vi "Main.vi"() -> ()   [LabVIEW 2017]
uses:
  Controles/Objetos.ctl
  <vilib>/addons/database/Connection.llb/Conn ObjectReference.ctl
  <vilib>/NI/AMC/Update Message Routing Info.vi
  <vilib>/NI/AMC/Create Multiple Messages.vi
  <vilib>/NI/AMC/Read Termination Message.vi
  <vilib>/NI/AMC/Create Single Message.vi
  <vilib>/NI/AMC/Send Message.vi
  <vilib>/NI/AMC/Globals.vi
  <vilib>/Utility/file.llb/Read Delimited Spreadsheet (string).vi
  Globals/Global.vi
  <vilib>/addons/database/Connection.llb/DB Tools Open Connec (Path).vi
  <vilib>/addons/database/_DB Variant To Data/Database Variant To Data.xnode
  <vilib>/addons/database/NI_Database_API.lvlib
  <vilib>/NI/AMC/AMC.lvlib
panel:
  out "BBDD":bool
  in  "Consulta":bool
  in  "Registrado":string
  in  "Cambiar de usuario":bool
  in  "Jiffy csv":path
  in  "Registrar":bool
  out "error out":errorcluster
  in  "Objetos":T1
  out "DataBase":bool
  # "Contabilizador"
  # "powered by"
  # "Contabilizador v01"
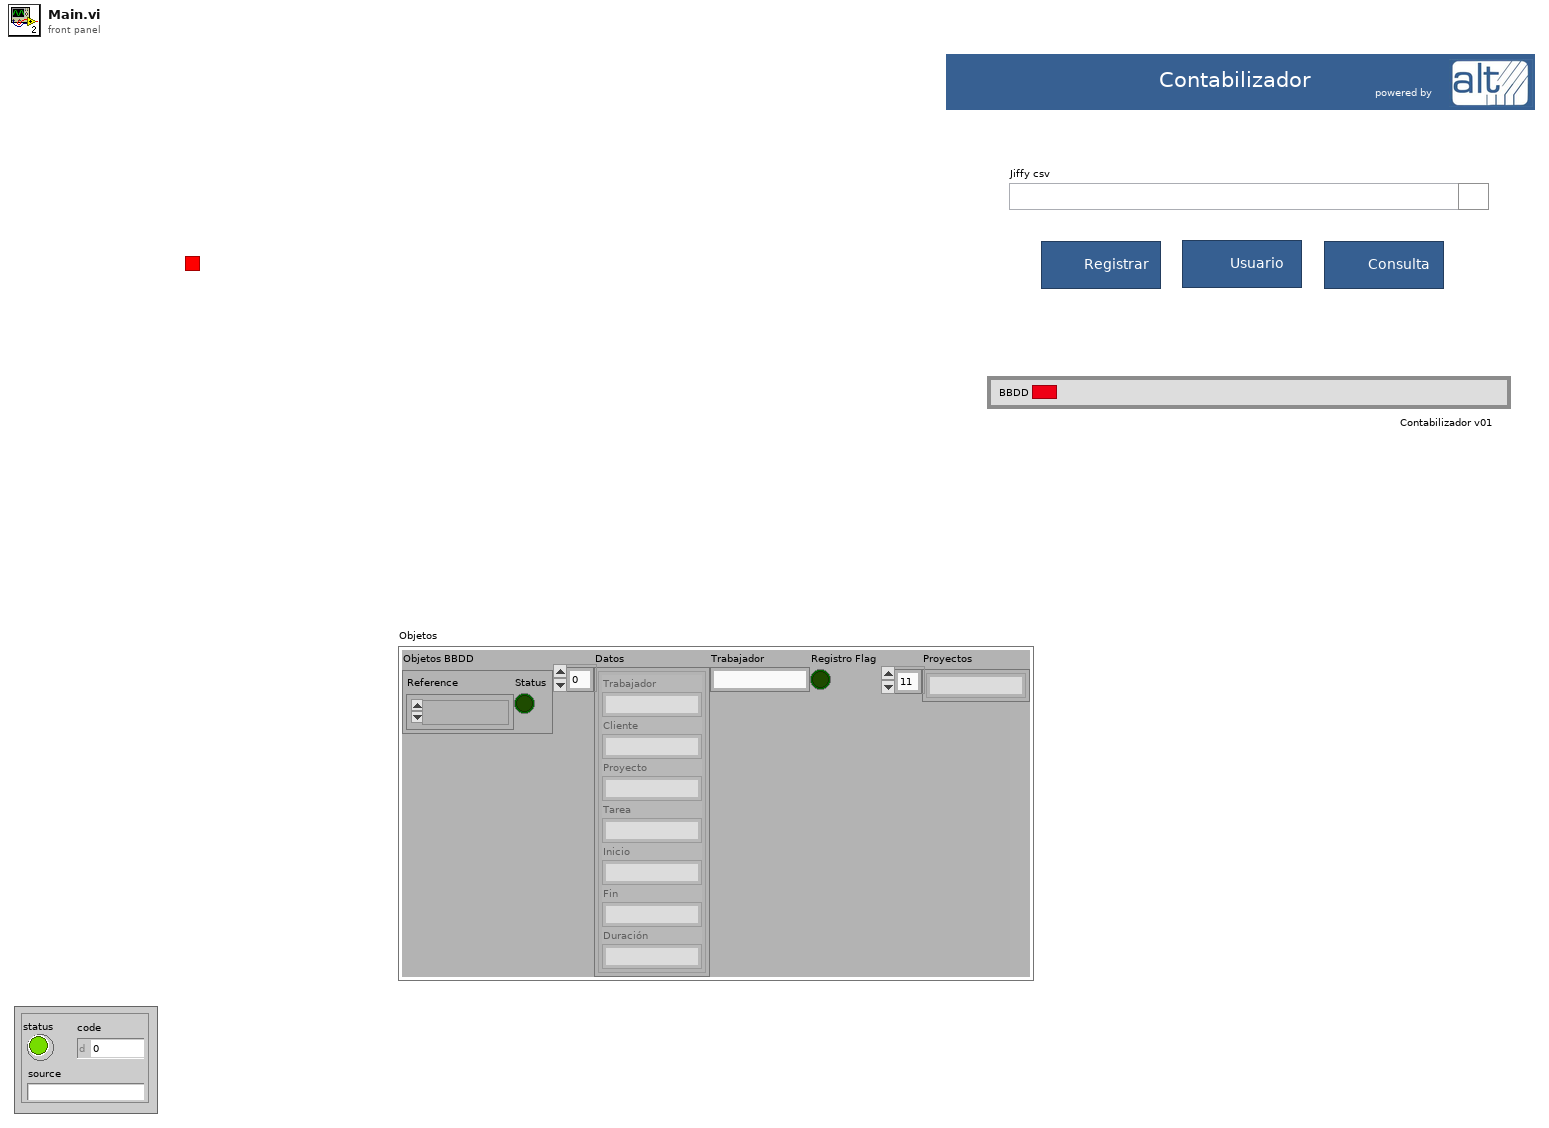
[diagram p1: front panel]
types:
  T1 = typedef "Objetos.ctl" = cluster{"Objetos BBDD":cluster{"Reference":T2, "Status":bool}, "Datos":cluster{"Trabajador":string, "Cliente":string, "Proyecto":string, "Tarea":string, "Inicio":string, "Fin":string, "Duración":string}[], "Trabajador":string, "Registro Flag":bool, "Proyectos":string[]}
  T2 = typedef "NI_Database_API.lvlib/Conn ObjectReference.ctl" = refnum<k1>
  T3 = typedef "AMC.lvlib/Message Queue.ctl" = refnum<queue>
  T4 = cluster{"Trabajador":string, "Cliente":string, "Proyecto":string, "Tarea":string, "Inicio":string, "Fin":string, "Duración":string}
  T5 = cluster{"Nombre de usuario":string, "Contraseña":string, "Trabajador":string}[]
  T6 = cluster{"Trabajador":string, "Cliente":string, "Proyecto":string, "Tarea":string, "Inicio":string, "Fin":string, "Duración":string}[]
  T7 = cluster{"Trabajador":string, "Cliente":string, "Proyecto":string, "Tarea":string, "Inicio":string, "Fin":string, i32}
  T8 = cluster{"Nombre":void, "Min":void, "Avg":void, "Max":void, "Condición":void, "Resultado":void, "date/time string":string}
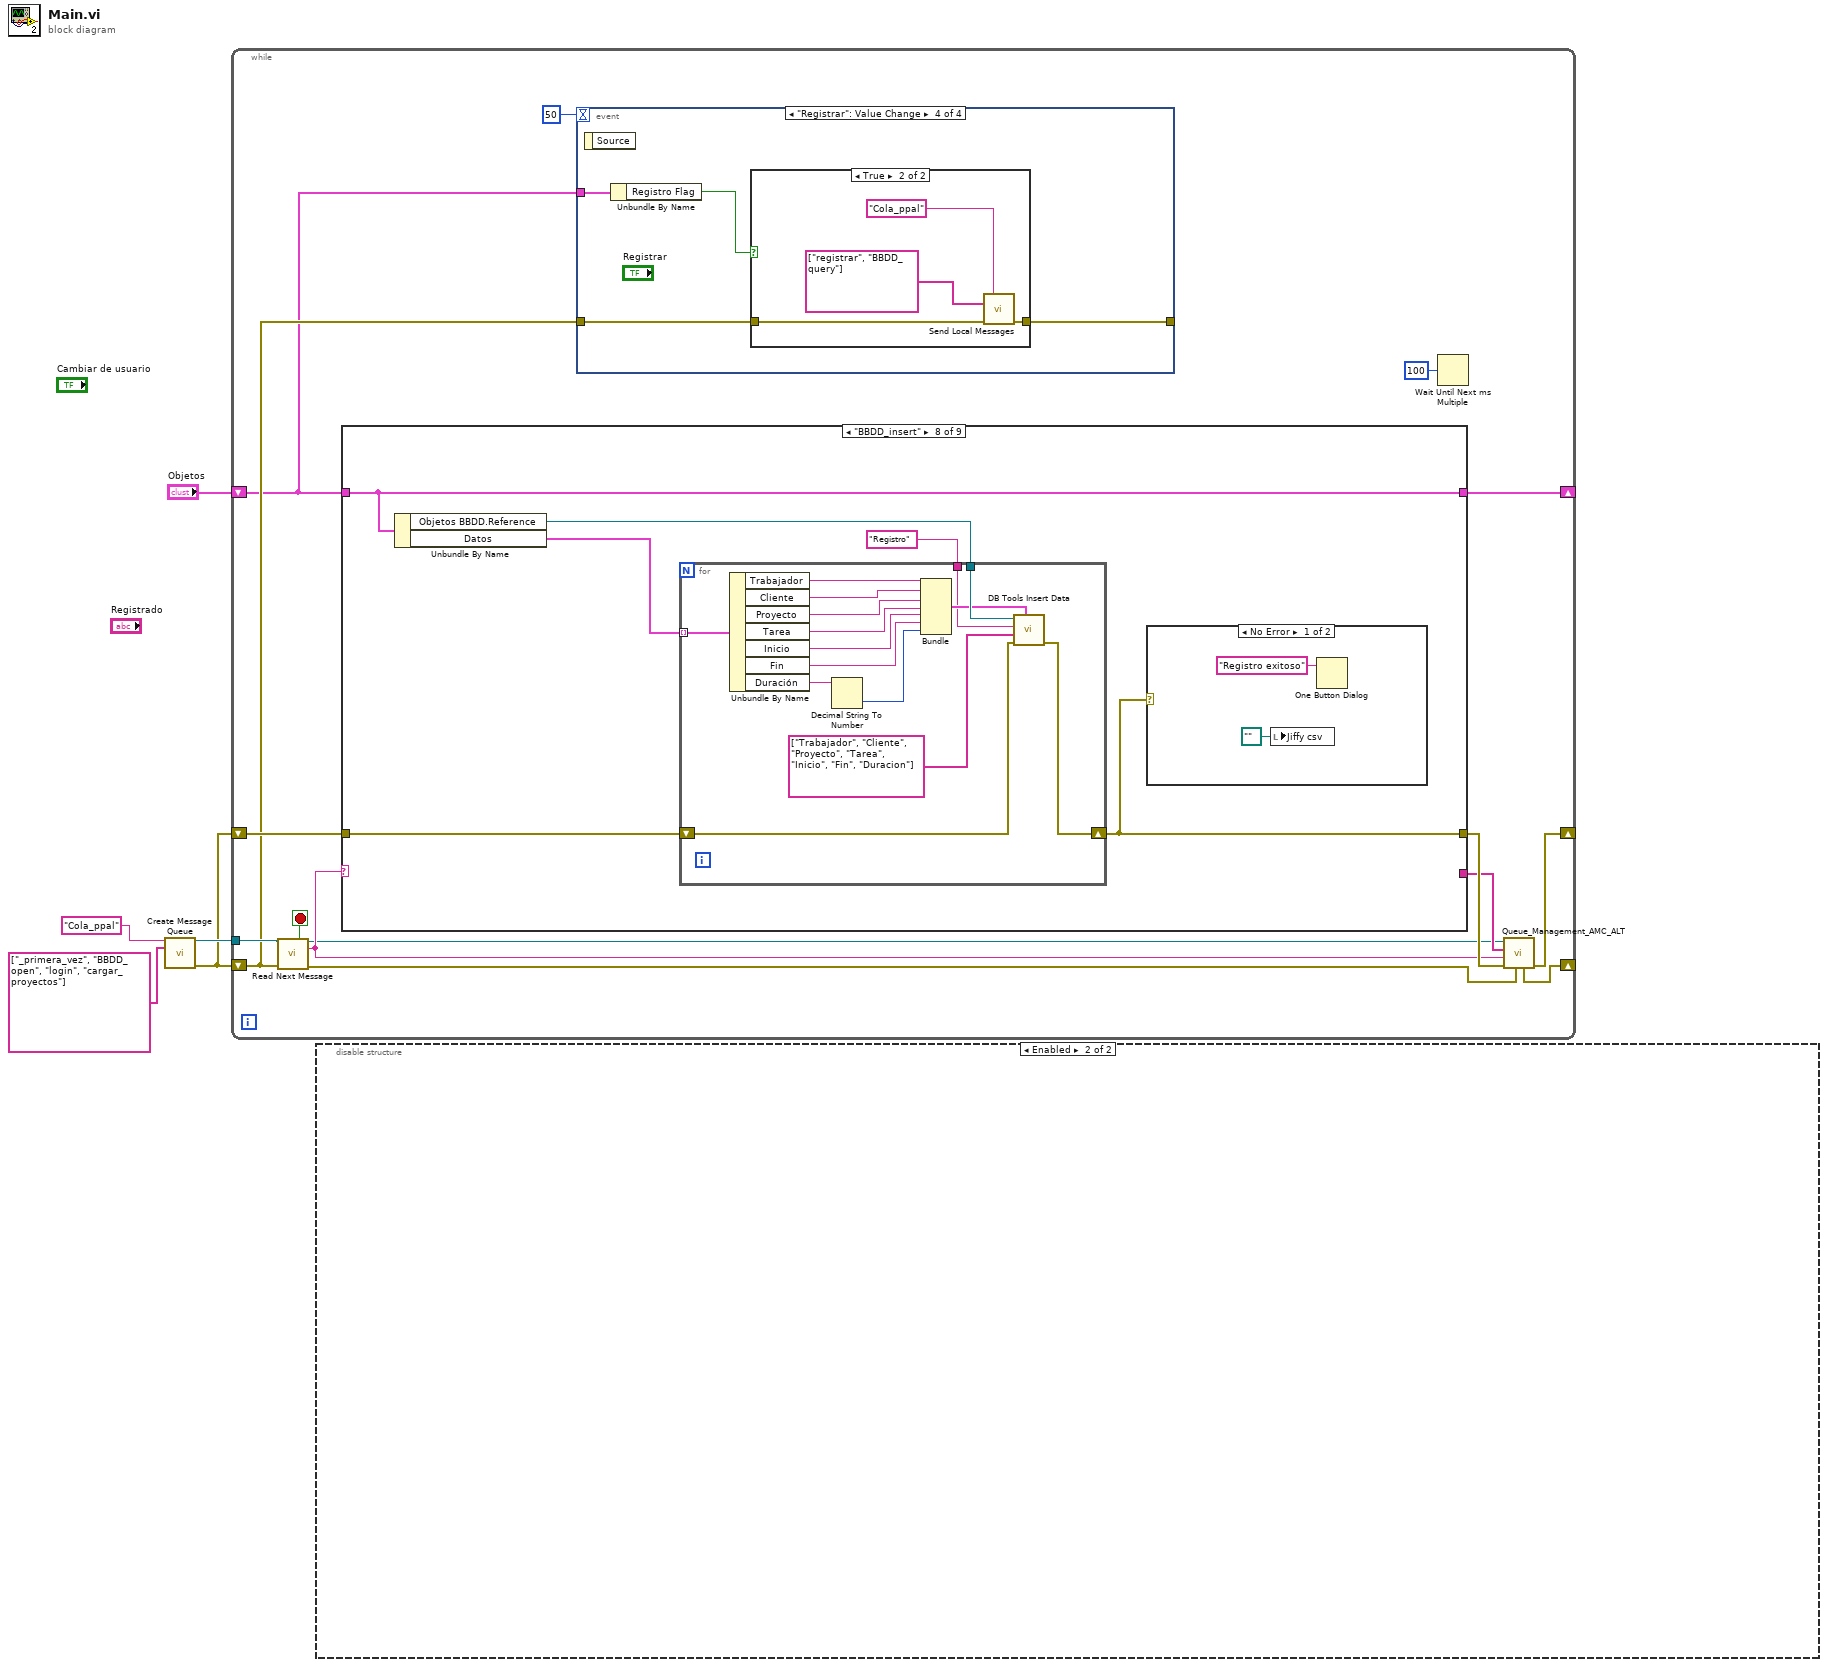
[diagram p0: block diagram]
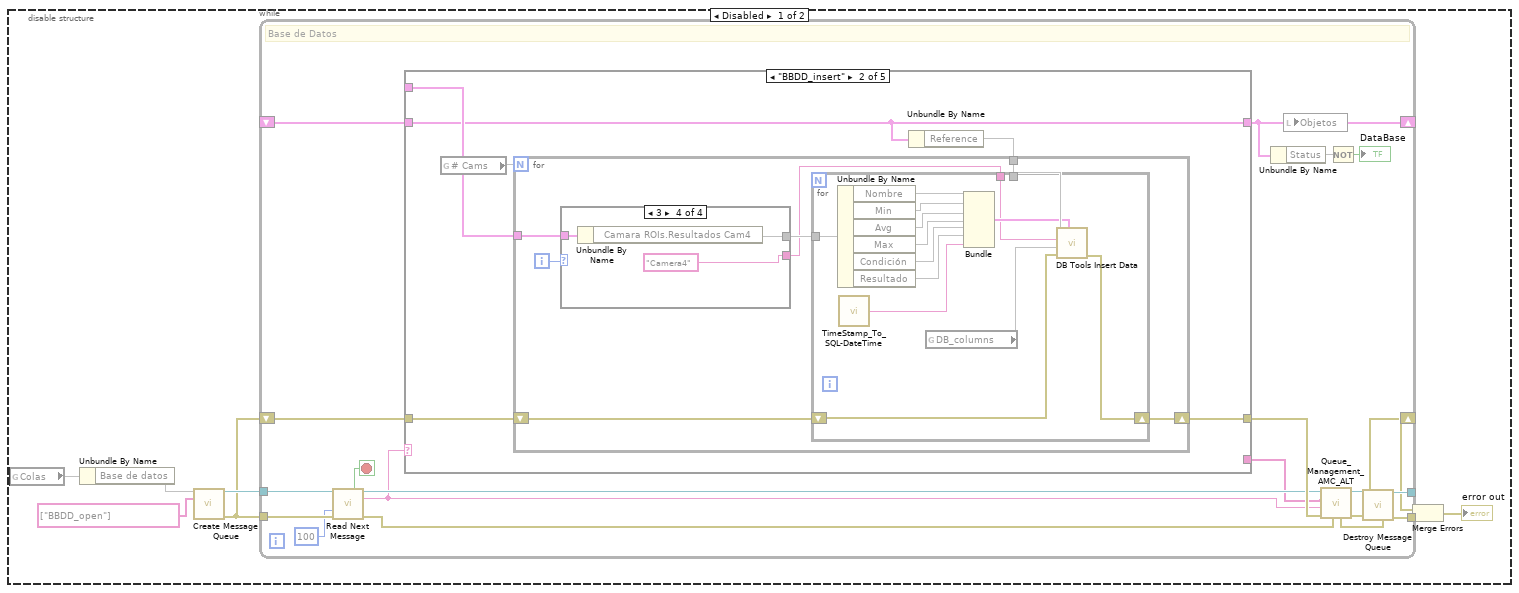
[diagram p2: hidden frame]
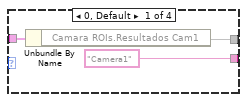
[diagram p4: hidden frame]
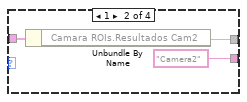
[diagram p5: hidden frame]
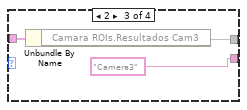
[diagram p6: hidden frame]
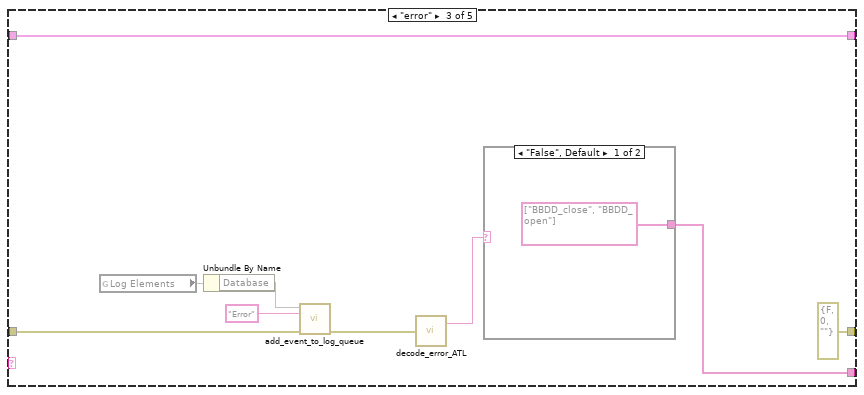
[diagram p7: hidden frame]
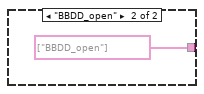
[diagram p8: hidden frame]
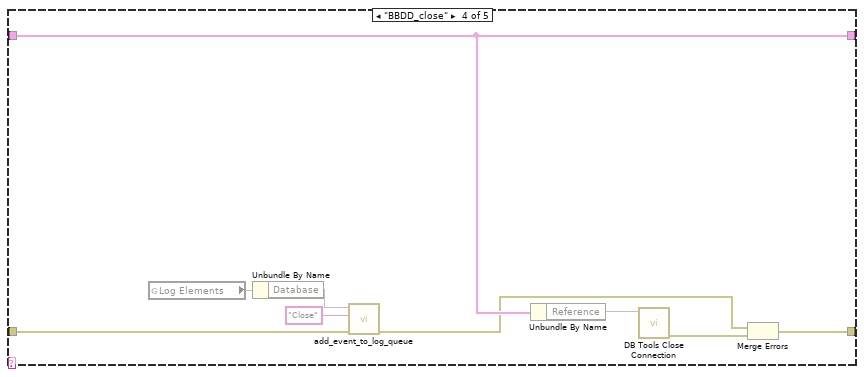
[diagram p9: hidden frame]
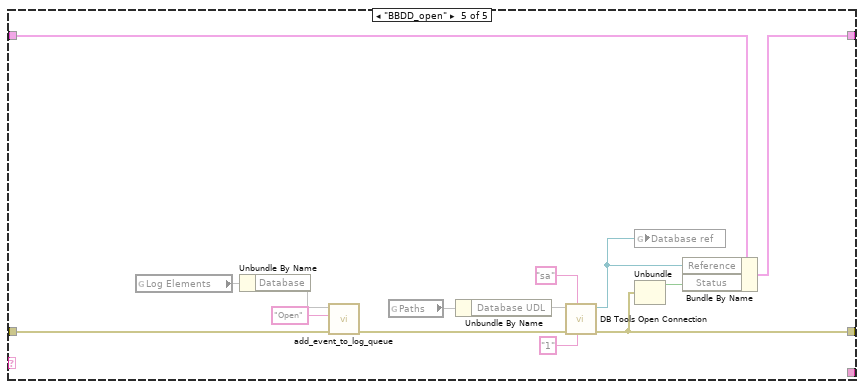
[diagram p10: hidden frame]
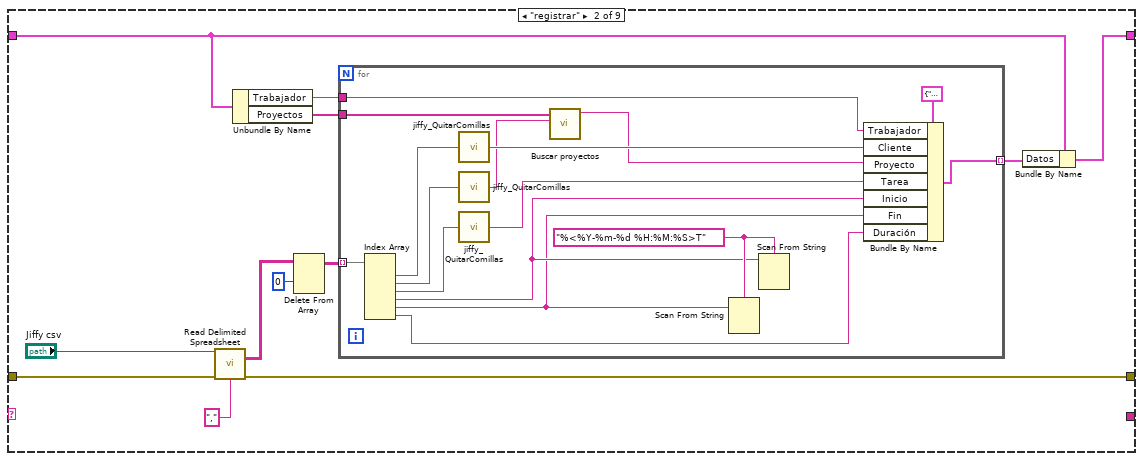
[diagram p12: hidden frame]
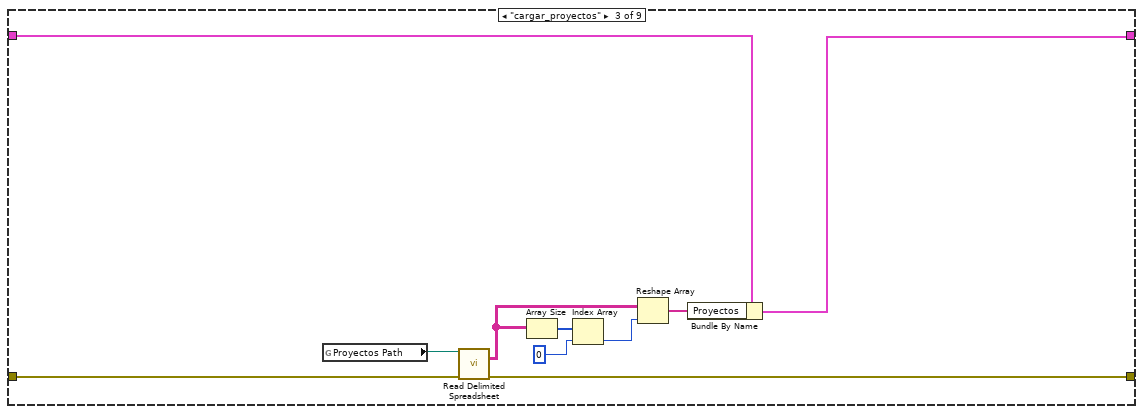
[diagram p13: hidden frame]
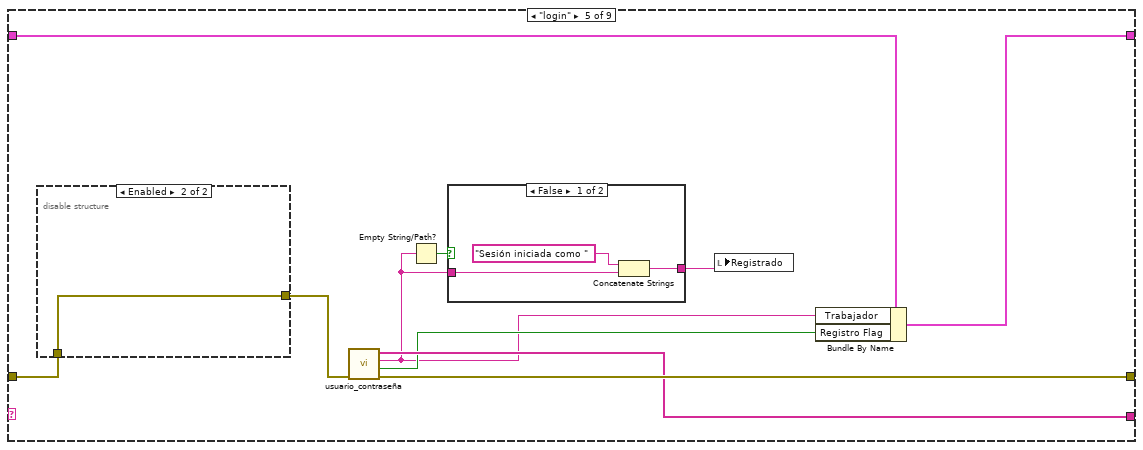
[diagram p15: hidden frame]
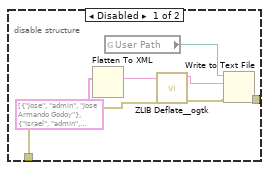
[diagram p16: hidden frame]
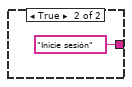
[diagram p17: hidden frame]
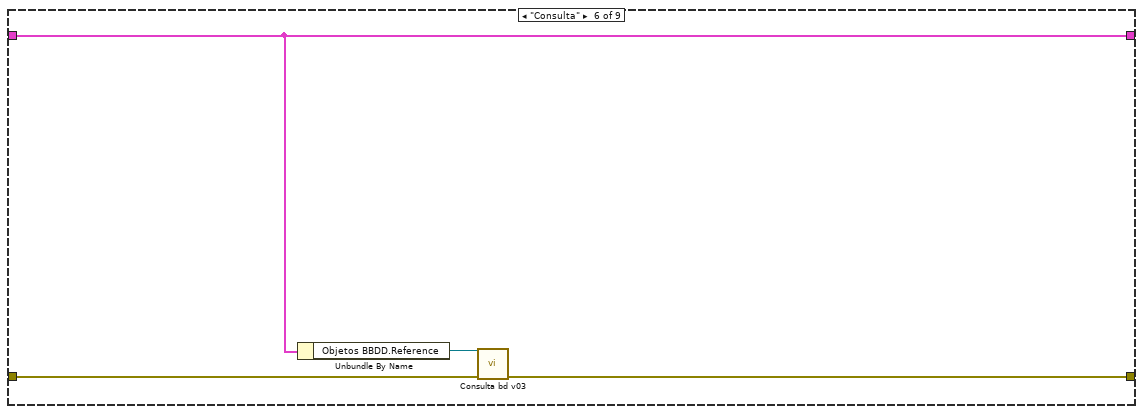
[diagram p18: hidden frame]
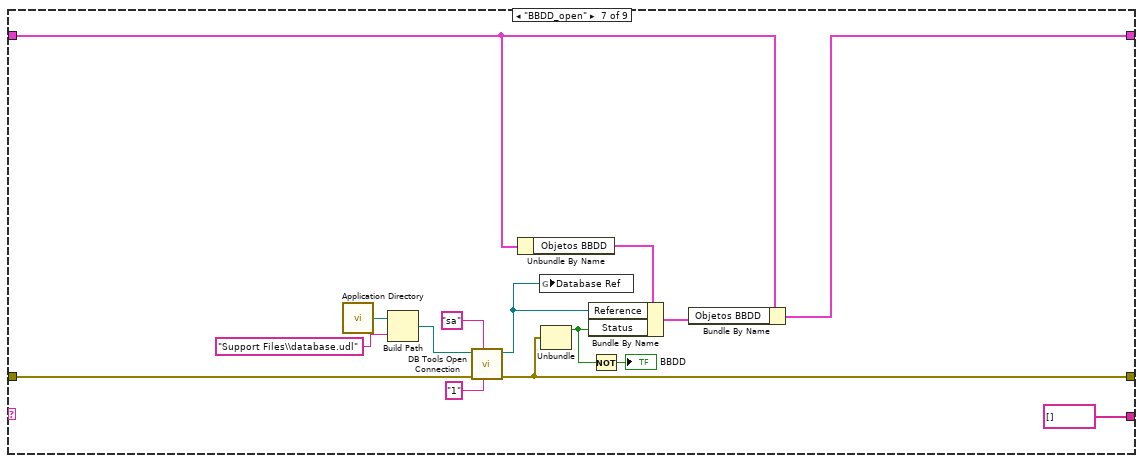
[diagram p19: hidden frame]
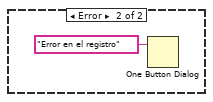
[diagram p20: hidden frame]
diagram:
  n1 = call <vilib>:"Create Message Queue.vi"("message queue name"="Cola_ppal", "initial message names"=string[] ["_primera_vez", "BBDD_open", "login", "cargar_proyectos"]) -> ("message queue out"=w4:T3, "error out"=w1:errorcluster)  [unwired: 12 in]
  n2 = while {
    shift-right: [w17] -> _
    shift-left: w1 -> [w9]
    tunnel: w4 -> [w19]
    shift-right: [w16] -> _
    shift-left: "Objetos" -> [w7]
    shift-right: [w13] -> _
    shift-left: w1 -> [w14]
    stop <- w20 stop-if-true
    n3 = call <vilib>:"Read Next Message.vi"("message queue in"=w19, "error in"=w9) -> ("exit process?"=w20:bool, "message queue out"=w10:T3, "message name"=w11:string, "error out"=w18:errorcluster)  [unwired: 6 in, 4 out]
    n4 = case shown="\"BBDD_insert\"" w11 {
      tunnel: w7 -> [w21 w29 w56 w61 w68 w85 w97 w107 w132]
      tunnel: [w21 w33 w55 w61 w67 w85 w96 w107 w131] -> w16
      tunnel: w14 -> [_ w32 w59 w60 w71 w87 w95 w108 w138]
      tunnel: [_ w31 w58 w60 w70 w86 w94 w103 w135] -> w15
      tunnel: [_ _ _ _ w66 _ string[] [] ("Elementos a cola") _ w129] -> w12
      frame "False", Default {
      }
      frame "registrar" {
        n5 = call-poly <vilib>:"Read Delimited Spreadsheet.vi"("file path (dialog if empty)"="Jiffy csv", "error in (no error)"=w32, "delimiter (\\t)"="," ("delimiter (\\t)")) -> ("all rows"=w27:string[][], "error out"=w31:errorcluster)  [unwired: 7 in, 4 out]
        n6 = Unbundle By Name(w29) -> ("Trabajador"=w23:string, "Proyectos"=w22:string[])
        n7 = Delete From Array(array=w27, index (row)=0) -> (array with subset deleted=w26:string[][])  [unwired: 2 in, 1 out]
        n8 = for {
          tunnel: w26 -> [w49] mode=indexing
          tunnel: [w39] -> w24 mode=indexing
          tunnel: w23 -> [w37]
          tunnel: w22 -> [w35]
          w46 = "%<%Y-%m-%d %H:%M:%S>T" ("format string")
          n9 = Index Array(array=w49) -> (element #1=w45:string, element #2=w48:string, element #3=w47:string, element #4=w41:string, element #5=w40:string, element #6=w38:string)  [unwired: 6 in]
          n10 = call "jiffy_QuitarComillas.vi"("String in"=w45) -> ("String out"=w43:string)
          n11 = call "jiffy_QuitarComillas.vi"("String in"=w48) -> ("String out"=w36:string)
          n12 = call "jiffy_QuitarComillas.vi"("String in"=w47) -> ("String out"=w42:string)
          n13 = call "Buscar proyectos.vi"("String out"=w36, "Proyectos"=w35) -> ("Proyecto"=w34:string)  [unwired: 9 in]
          n14 = Scan From String(format string=w46, input string=w40) -> ()  [unwired: 4 in, 3 out]
          n15 = Scan From String(format string=w46, input string=w41) -> ()  [unwired: 4 in, 3 out]
          n16 = Bundle By Name(cluster=T4 {"Trabajador"="", "Cliente"="", "Proyecto"="", "Tarea"="", "Inicio"="", "Fin"="", "Duración"=""} ("Cluster"), "Trabajador"=w37, "Cliente"=w43, "Proyecto"=w34, "Tarea"=w42, "Inicio"=w41, "Fin"=w40, "Duración"=w38) -> (w39:T4)
        }
        n17 = Bundle By Name(cluster=w29, "Datos"=w24) -> (w33:T1)
      }
      frame "cargar_proyectos" {
        n18 = global read "Global.vi" "Proyectos Path"() -> (w57:path)
        n19 = call-poly <vilib>:"Read Delimited Spreadsheet.vi"("file path (dialog if empty)"=w57, "error in (no error)"=w59) -> ("all rows"=w53:string[][], "error out"=w58:errorcluster)  [unwired: 8 in, 4 out]
        n20 = Array Size(array=w53) -> (size(s)=w52:i32[])
        n21 = Index Array(array=w52, index=0) -> (element=w50:i32)
        n22 = Reshape Array(w53, w50) -> (w54:string[])
        n23 = Bundle By Name(cluster=w56, "Proyectos"=w54) -> (w55:T1)
      }
      frame "_primera_vez" {
      }
      frame "login" {
        n24 = disable-structure shown="Enabled" {
          disable-tunnel: w71 -> [w78 w79]
          disable-tunnel: [w77 w79] -> w69
          frame Disabled {
            n25 = Flatten To XML(anything=T5 [{"Nombre de usuario"="Jose", "Contraseña"="admin", "Trabajador"="Jose Armando Godoy"}, {"Nombre de usuario"="Israel", "Contraseña"="admin", "Trabajador"="Israel Garcia"}, {"Nombre de usuario"="Alejandro", "Contraseña"="admin", "Trabajador"="Alejandro Ortiz"}, {"Nombre de usuario"="Jair", "Contraseña"="admin", "Trabajador"="Jair Paredes"}] ("Array")) -> (xml string=w73:string)
            n26 = global read "Global.vi" "User Path"() -> (w72:path)
            n27 = call <userlib>:"ZLIB Deflate__ogtk.vi"("error in (no error)"=w78, "input"=w73) -> ("error out"=w75:errorcluster, "deflated output"=w76:string)  [unwired: 3 in, 1 out]
            n28 = Write to Text File(file (use dialog)=w72, text=w76, error in=w75) -> (error out=w77:errorcluster)  [unwired: 1 in, 2 out]
          }
          frame Enabled {
          }
        }
        n29 = call "usuario_contraseña.vi"("error in"=w69) -> ("error out"=w70:errorcluster, "Registro Flag"=w65:bool, "Trabajador"=w62:string, "Elemento a cola"=w66:string[])  [unwired: 7 in]
        n30 = Empty String/Path?(string/path=w62) -> (empty?=w64:bool)
        n31 = case shown="False" w64 {
          tunnel: [w81 "Inicie sesión"] -> w63
          tunnel: w62 -> [w80 _]
          frame False {
            n32 = Concatenate Strings("Sesión iniciada como ", w80) -> (w81:string)
          }
          frame True {
          }
        }
        n33 = local write "Registrado"(w63) -> ()
        n34 = Bundle By Name(cluster=w68, "Trabajador"=w62, "Registro Flag"=w65) -> (w67:T1)
      }
      frame "Consulta" {
        n35 = Unbundle By Name(w85) -> ("Objetos BBDD.Reference"=w84:T2)
        n36 = call "Consulta bd v03.vi"("error in (no error)"=w87, "Database"=w84) -> ("error out"=w86:errorcluster)  [unwired: 9 in]
      }
      frame "BBDD_open" {
        n37 = call <vilib>:"Application Directory.vi"() -> ("Application Directory"=w93:path)
        n38 = Build Path(base path=w93, name or relative path="Support Files\\database.udl") -> (appended path=w91:path)
        n39 = call-poly <vilib>:"DB Tools Open Connection.vi"("password"="1", "userID"="sa", "error in (no error)"=w95, "connection information"=w91) -> ("error out"=w94:errorcluster, "connection reference"=w88:T2)  [unwired: 4 in]
        n40 = Unbundle By Name(w97) -> ("Objetos BBDD"=w99:cluster{"Reference":T2, "Status":bool})
        n41 = global write "Global.vi" "Database Ref"(w88) -> ()
        n42 = Unbundle(w94) -> ("status"=w100:bool)  [unwired: 2 out]
        n43 = Bundle By Name(cluster=w99, "Reference"=w88, "Status"=w100) -> (w98:cluster{"Reference":T2, "Status":bool})
        n44 = Not(x=w100) -> (.not. x?=→"BBDD":bool)
        n45 = Bundle By Name(cluster=w97, "Objetos BBDD"=w98) -> (w96:T1)
      }
      frame "BBDD_insert" {
        n46 = Unbundle By Name(w107) -> ("Objetos BBDD.Reference"=w105:T2, "Datos"=w106:T6)
        n47 = for {
          tunnel: w106 -> [w126] mode=indexing
          tunnel: w105 -> [w124]
          shift-right: [w117] -> w103
          shift-left: w108 -> [w118]
          tunnel: "Registro" ("table") -> [w115]
          n48 = Unbundle By Name(w126) -> ("Trabajador"=w125:string, "Cliente"=w119:string, "Proyecto"=w120:string, "Tarea"=w121:string, "Inicio"=w122:string, "Fin"=w116:string, "Duración"=w114:string)
          n49 = Decimal String To Number(string=w114) -> (number=w113:i32)  [unwired: 2 in, 1 out]
          n50 = Bundle("Trabajador"=w125, "Cliente"=w119, "Proyecto"=w120, "Tarea"=w121, "Inicio"=w122, "Fin"=w116, w113) -> (w123:T7)  [unwired: 1 in]
          n51 = call <vilib>:"DB Tools Insert Data.vi"("data"=w123, "error in (no error)"=w118, "columns"=string[] ["Trabajador", "Cliente", "Proyecto", "Tarea", "Inicio", "Fin", "Duracion"], "table"=w115, "connection reference"=w124) -> ("error out"=w117:errorcluster)  [unwired: 5 in, 1 out]
        }
        n52 = case shown="No Error" w103 {
          frame No Error {
            n53 = local write "Jiffy csv"(path "" ("Jiffy csv")) -> ()
            n54 = One Button Dialog(message="Registro exitoso") -> ()  [unwired: 1 in, 1 out]
          }
          frame Error {
            n55 = One Button Dialog(message="Error en el registro") -> ()  [unwired: 1 in, 1 out]
          }
        }
      }
      frame "BBDD_query" {
        # "Selecciona que lineas del archivo se guardaran.\nSi la linea ha sido guardada entonces no se duplica"
        n56 = Unbundle By Name(w132) -> ("Objetos BBDD.Reference"=w136:T2, "Datos"=w137:T6)
        n57 = for {
          tunnel: w137 -> [w143] mode=indexing
          tunnel: w136 -> [w151]
          shift-right: [w146] -> w135
          shift-left: w138 -> [w152]
          tunnel: " \nWHERE Inicio >= Convert(datetime,'%s',111)\nAND Fin <= Convert(datetime,'%s',111)\nAND Proyecto ='%s'\nAND Trabajador ='%s'\nAND Tarea ='%s'" ("condition") -> [w159]
          tunnel: "Registro" ("table") -> [w150]
          tunnel: [w143] -> w130 mode=indexing if=w142
          tunnel: [w142] -> w128 mode=indexing
          n58 = Unbundle By Name(w143) -> ("Trabajador"=w155:string, "Proyecto"=w156:string, "Tarea"=w154:string, "Inicio"=w158:string, "Fin"=w157:string)
          n59 = Format Into String(format string=w159, w158, w157, w156, w155, w154) -> (resulting string=w153:string)  [unwired: 2 in, 1 out]
          n60 = call <vilib>:"DB Tools Select Data.vi"("condition"=w153, "error in (no error)"=w152, "columns"=string[] ["Trabajador"], "table"=w150, "connection reference"=w151) -> ("error out"=w147:errorcluster, "data"=w148:variant[][])  [unwired: 1 in, 1 out]
          n61 = xnode "Database Variant To Data"("database variant"=w148, "error in (no error)"=w147, "type"=cluster{"Trabajador":string}[] []) -> ("data"=w144:cluster{"Trabajador":string}[], "error out"=w146:errorcluster)
          n62 = Empty Array?(array=w144) -> (empty?=w142:bool)
        }
        n63 = Or Array Elements(Boolean array=w128) -> (logical OR=w127:bool)
        n64 = Bundle By Name(cluster=w132, "Datos"=w130) -> (w131:T1)
        n65 = case shown="True" w127 {
          tunnel: [_ string[] ["BBDD_insert"] ("message name")] -> w129
          frame False {
            n66 = local write "Jiffy csv"(path "" ("Jiffy csv")) -> ()
            n67 = One Button Dialog(message="Este archivo ya ha sido guardado con anterioridad") -> ()  [unwired: 1 in, 1 out]
          }
          frame True {
          }
        }
      }
    }
    n68 = event shown="[3] \"Registrar\": Value Change" {
      selector: _ -> [_ _ _ _]
      dyn-events: _ -> [_ _ _ _]
      timeout: 50 -> [_ _ _ _]
      tunnel: w9 -> [w201 w202 w207 w213]
      tunnel: [w201 w203 w206 w212] -> _
      tunnel: w7 -> [_ _ _ w211]
      event Timeout {
        n69 = event-data() -> ()  [unwired: 1 in, 3 out]
      }
      event "Consulta": Mouse Up {
        n70 = event-data() -> ()  [unwired: 1 in, 1 out]
        n71 = call <vilib>:"Send Local Messages.vi"("receiver process (\"\" - local)"="Cola_ppal" ("receiver process (\"\" - local)"), "message names"=string[] ["Consulta"] ("message name"), "error in"=w202) -> ("error out"=w203:errorcluster)  [unwired: 10 in, 2 out]
      }
      event "Cambiar de usuario": Mouse Up {
        n72 = event-data() -> ()  [unwired: 1 in, 8 out]
        n73 = call <vilib>:"Send Local Messages.vi"("receiver process (\"\" - local)"="Cola_ppal" ("receiver process (\"\" - local)"), "message names"=string[] ["login"] ("message name"), "error in"=w207) -> ("error out"=w206:errorcluster)  [unwired: 10 in, 2 out]
      }
      event "Registrar": Value Change {
        n74 = event-data() -> ()  [unwired: 1 in, 1 out]
        n75 = Unbundle By Name(w211) -> ("Registro Flag"=w210:bool)
        n76 = case shown="True" w210 {
          tunnel: w213 -> [w215 w218]
          tunnel: [w215 w217] -> w212
          frame False {
            n77 = One Button Dialog(message="Inicie sesión") -> ()  [unwired: 1 in, 1 out]
          }
          frame True {
            n78 = call <vilib>:"Send Local Messages.vi"("receiver process (\"\" - local)"="Cola_ppal" ("receiver process (\"\" - local)"), "message names"=string[] ["registrar", "BBDD_query"] ("message name"), "error in"=w218) -> ("error out"=w217:errorcluster)  [unwired: 10 in, 2 out]
          }
        }
      }
    }
    n79 = Wait Until Next ms Multiple(millisecond multiple=u32 100) -> ()  [unwired: 1 out]
    n80 = call "Queue_Management_AMC_ALT.vi"("queue error in"=w18, "system error in"=w15, "Case"=w11, "Elementos a cola"=w12, "message queue in"=w10) -> ("system error out"=w13:errorcluster, "queue error out"=w17:errorcluster)  [unwired: 3 in, 2 out]
  }
  n81 = disable-structure shown="Enabled" {
    frame Disabled {
      n82 = global read "Global.vi" "Colas"() -> (w221)
      n83 = Unbundle By Name(w221) -> ("Base de datos"=w220)
      n84 = call <vilib>:"Create Message Queue.vi"("message queue name"=w220, "initial message names"=string[] ["BBDD_open"]) -> ("message queue out"=w228:T3, "error out"=w227:errorcluster)  [unwired: 12 in]
      n85 = while {
        tunnel: w228 -> [w246]
        tunnel: w227 -> [w245]
        shift-right: [w233] -> _
        shift-left: _ -> [w243]
        shift-right: [w241] -> w223
        shift-left: w227 -> [w244]
        tunnel: [w236] -> w226
        tunnel: [w235] -> w225
        stop <- w230 stop-if-true
        # "Base de Datos"
        n86 = call <vilib>:"Read Next Message.vi"("message queue in"=w246, "timeout (1 ms)"=100, "error in"=w245) -> ("exit process?"=w230:bool, "message queue out"=w239:T3, "message name"=w237:string, "error out"=w238:errorcluster)  [unwired: 5 in, 4 out]
        n87 = case shown="\"BBDD_insert\"" w237 {
          tunnel: w244 -> [w247 w253 w292 w302 w314]
          tunnel: w243 -> [w248 w250 w295 w306 w319]
          tunnel: [w248 w250 w295 w306 w318] -> w233
          tunnel: [w247 w252 errorcluster {"status"=FALSE, "code"=0, "source"=""} ("error out") w304 w315] -> w240
          tunnel: _ -> [_ w251 _ _ _]
          tunnel: [_ _ w293 _ _] -> w234
          frame "Timeout", Default {
          }
          frame "BBDD_insert" {
            n88 = global read "Global.vi" "# Cams"() -> (w249)
            n89 = Unbundle By Name(w250) -> ("Reference"=w254)
            n90 = for {
              N: w249 -> [_]
              tunnel: w254 -> [w261]
              shift-right: [w259] -> w252
              shift-left: w253 -> [w260]
              tunnel: w251 -> [w256]
              i -> [w258]
              n91 = case shown="3" w258 {
                tunnel: [w264 w267 w270 w273] -> w257
                tunnel: w256 -> [w263 w266 w269 w272]
                tunnel: ["Camera1" ("table") "Camera2" ("table") "Camera3" ("table") "Camera4" ("table")] -> w255
                frame 0, Default {
                  n92 = Unbundle By Name(w263) -> ("Camara ROIs.Resultados Cam1"=w264)
                }
                frame 1 {
                  n93 = Unbundle By Name(w266) -> ("Camara ROIs.Resultados Cam2"=w267)
                }
                frame 2 {
                  n94 = Unbundle By Name(w269) -> ("Camara ROIs.Resultados Cam3"=w270)
                }
                frame 3 {
                  n95 = Unbundle By Name(w272) -> ("Camara ROIs.Resultados Cam4"=w273)
                }
              }
              n96 = for {
                tunnel: w257 -> [w287]
                tunnel: w261 -> [w285]
                shift-right: [w278] -> w259
                shift-left: w260 -> [w279]
                tunnel: w255 -> [w275]
                n97 = Unbundle By Name(w287) -> ("Nombre"=w286, "Min"=w280, "Avg"=w281, "Max"=w282, "Condición"=w283, "Resultado"=w277)
                n98 = call "TimeStamp_To_SQL-DateTime.vi"() -> ("date/time string"=w276:string)  [unwired: 1 in]
                n99 = global read "Global.vi" "DB_columns"() -> (w274)
                n100 = Bundle("Nombre"=w286, "Min"=w280, "Avg"=w281, "Max"=w282, "Condición"=w283, "Resultado"=w277, "date/time string"=w276) -> (w284:T8)  [unwired: 1 in]
                n101 = call <vilib>:"DB Tools Insert Data.vi"("data"=w284, "error in (no error)"=w279, "columns"=w274, "table"=w275, "connection reference"=w285) -> ("error out"=w278:errorcluster)  [unwired: 5 in, 1 out]
              }
            }
          }
          frame "error" {
            n102 = global read "Global.vi" "Log Elements"() -> (w290)
            n103 = Unbundle By Name(w290) -> ("Database"=w289)
            n104 = call "add_event_to_log_queue.vi"("error in (no error)"=w292, "Evento"="Error", "Elemento"=w289) -> ("error out"=w291:errorcluster)  [unwired: 8 in]
            n105 = call "decode_error_ATL.vi"("error in (no error)"=w291) -> ("case"=w294:string)  [unwired: 1 out]
            n106 = case shown="\"False\", Default" w294 {
              tunnel: [string[] ["BBDD_close", "BBDD_open"] ("message names") string[] ["BBDD_open"] ("message names")] -> w293
              frame "False", Default {
              }
              frame "BBDD_open" {
              }
            }
          }
          frame "BBDD_close" {
            n107 = global read "Global.vi" "Log Elements"() -> (w303)
            n108 = Unbundle By Name(w303) -> ("Database"=w300)
            n109 = call "add_event_to_log_queue.vi"("error in (no error)"=w302, "Evento"="Close", "Elemento"=w300) -> ("error out"=w301:errorcluster)  [unwired: 8 in]
            n110 = Unbundle By Name(w306) -> ("Reference"=w307)
            n111 = call <vilib>:"DB Tools Close Connection.vi"("connection reference"=w307) -> ("error out"=w305:errorcluster)  [unwired: 6 in]
            n112 = Merge Errors(w301, w305) -> (w304:errorcluster)
          }
          frame "BBDD_open" {
            n113 = global read "Global.vi" "Log Elements"() -> (w312)
            n114 = Unbundle By Name(w312) -> ("Database"=w309)
            n115 = call "add_event_to_log_queue.vi"("error in (no error)"=w314, "Evento"="Open", "Elemento"=w309) -> ("error out"=w313:errorcluster)  [unwired: 8 in]
            n116 = global read "Global.vi" "Paths"() -> (w311)
            n117 = Unbundle By Name(w311) -> ("Database UDL"=w310)
            n118 = call-poly <vilib>:"DB Tools Open Connection.vi"("password"="1", "userID"="sa", "error in (no error)"=w313, "connection information"=w310) -> ("error out"=w315:errorcluster, "connection reference"=w316:T2)  [unwired: 4 in]
            n119 = global write "Global.vi" "Database ref"(w316) -> ()
            n120 = Unbundle(w315) -> ("status"=w317:bool)  [unwired: 2 out]
            n121 = Bundle By Name(cluster=w319, "Reference"=w316, "Status"=w317) -> (w318:cluster{})
          }
        }
        n122 = Unbundle By Name(w233) -> ("Status"=w232)
        n123 = local write "Objetos"(w233) -> ()
        n124 = call "Queue_Management_AMC_ALT.vi"("queue error in"=w238, "system error in"=w240, "Case"=w237, "Elementos a cola"=w234, "message queue in"=w239) -> ("system error out"=w241:errorcluster, "message queue out"=w236:T3, "queue error out"=w235:errorcluster)  [unwired: 3 in, 1 out]
        n125 = Not(x=w232) -> (.not. x?=→"DataBase":bool)
      }
      n126 = call <vilib>:"Destroy Message Queue.vi"("message queue in"=w226, "error in"=w225) -> ("error out"=w224:errorcluster)  [unwired: 11 in, 2 out]
      n127 = Merge Errors(w223, w224) -> (→"error out":errorcluster)
    }
    frame Enabled {
    }
  }
